vi "Write Configuration.vi"(8 "error in":errorcluster, 10 "1553 channels":T2[](array[typedef]), 11 "Ballard MIL-STD 1553 custom device in":T1 format="%.0x") -> (0 "error out":errorcluster, 3 "Ballard MIL-STD 1553 custom device out":T1 format="%.0x")   [LabVIEW 2020, in "Ballard MIL-STD-1553 Scripting.lvlib"]
uses:
  Ballard MIL-STD-1553 Scripting.lvlib
  <vilib>/NI VeriStand/Custom Device API/Custom Device Item Ref.ctl
  Shared/1553 Channel.ctl
  Shared/Address.ctl
  Shared/Message Definition.ctl
  Shared/Message Type.ctl
  Shared/Terminal Endpoint.ctl
  Shared/Parameter Definition.ctl
  <vilib>/NI VeriStand/Custom Device API/Custom Device API.lvlib
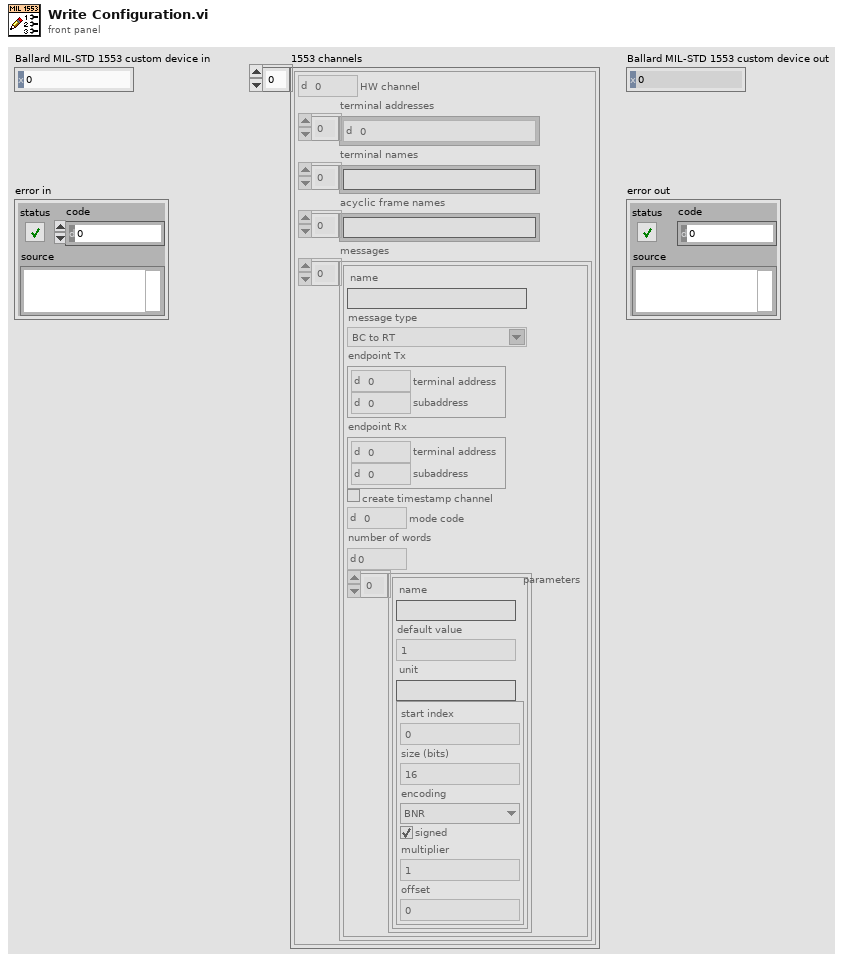
[diagram p1: front panel]
types:
  T1 = typedef "Custom Device API.lvlib/Custom Device Item Ref.ctl" = u64
  T2 = typedef "1553 Channel.ctl" = cluster{"HW channel":u16, "terminal addresses":T3[], "terminal names":string[], "acyclic frame names":string[], "messages":T4[]}
  T3 = typedef "Address.ctl" = u16
  T4 = typedef "Message Definition.ctl" = cluster{"name":string, "message type":T5, "endpoint Tx":T6, "endpoint Rx":T6, "create timestamp channel":bool, "mode code":u16, "number of words":u16, "parameters":cluster{"name":string, "default value":dbl, "unit":string, "parameter definition":T7}[]}
  T5 = typedef "Message Type.ctl" = string
  T6 = typedef "Terminal Endpoint.ctl" = cluster{"terminal address":T3, "subaddress":T3}
  T7 = typedef "Parameter Definition.ctl" = cluster{"start index":i32, "size (bits)":i32, "encoding":enum16{"BNR", "BCD", "Discrete"}, "signed":bool, "multiplier":dbl, "offset":dbl}
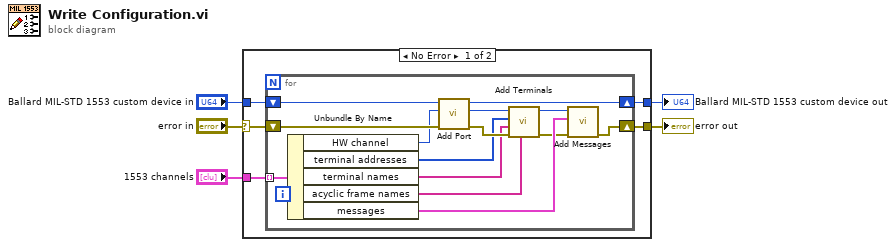
[diagram p0: block diagram]
diagram:
  n1 = case shown="No Error" "error in" {
    selector: "error in" -> [w7 w25]
    tunnel: [w10 w25] -> w5
    tunnel: [w9 w26] -> w4
    tunnel: "1553 channels" -> [w8 _]
    tunnel: "Ballard MIL-STD 1553 custom device in" -> [w6 w26]
    frame No Error {
      n2 = for {
        shift-right: [w20] -> w9
        shift-left: w6 -> [w23]
        tunnel: w8 -> [w24] mode=indexing
        shift-right: [w18] -> w10
        shift-left: w7 -> [w22]
        n3 = Unbundle By Name(w24) -> ("HW channel"=w21:u16, "terminal addresses"=w13:T3[], "terminal names"=w11:string[], "acyclic frame names"=w12:string[], "messages"=w19:T4[])
        n4 = call "Add Port.vi"("error in"=w22, "port number"=w21, "Ballard MIL-STD 1553 custom device in"=w23) -> ("error out"=w16:errorcluster, "port"=w17:T1, "Ballard MIL-STD 1553 custom device out"=w20:T1)  [unwired: 6 in]
        n5 = call "Add Terminals.vi"("acyclic frame names"=w12, "error in"=w16, "terminal names"=w11, "terminal addresses"=w13, "port in"=w17) -> ("error out"=w14:errorcluster, "port out"=w15:T1)  [unwired: 5 in]
        n6 = call "Add Messages.vi"("error in"=w14, "messages"=w19, "port in"=w15) -> ("error out"=w18:errorcluster)  [unwired: 7 in, 1 out]
      }
    }
    frame Error {
    }
  }
  "error out" <- w5
  "Ballard MIL-STD 1553 custom device out" <- w4
